vi "File Settings Dialog.vi"(8 "error in":errorcluster, 11 "Report Viewer in":refnum<class "Report Viewer.lvclass">) -> (0 "error out":errorcluster, 3 "Report Viewer out":refnum<class "Report Viewer.lvclass">)   [LabVIEW 2019, in "Report Viewer.lvlib" / "Report Viewer.lvclass"]
uses:
  Library/Report Viewer.lvclass
  Custom Controls/File Viewer Settings.ctl
  Custom Controls/Data Window.ctl
  Library/Report Viewer.lvclass/Report Viewer.ctl
  Custom Controls/Load Method.ctl
panel:
  in  "Default":bool caption="Cancel"
  in  "Cancel":bool
  in  "OK":bool caption="OK2"
  in  "File Navigation":enum32{"Number of Values", "By Time"}(tab)
  in  "Number of Values (graph)":T1={"Value Load"=enum."Load Selected", "Starting At"=0, "Number of Values"=100000}
  in  "Number of Values (table)":T1={"Value Load"=enum."Load Selected", "Starting At"=0, "Number of Values"=1000}
  in  "Data Window":T2 {"Seconds" max=60}
  # "Warning!  Setting the number of records too \nhigh can result in poor system performance"
  # "Warning!  Setting the number of records too \nhigh can result in poor system performance"
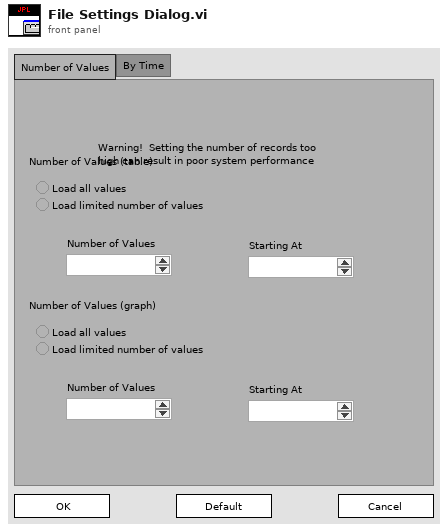
[diagram p1: front panel]
types:
  T1 = typedef "Report Viewer.lvlib/Report Viewer.lvclass/File Viewer Settings.ctl" = cluster{"Value Load":enum32{"Load All", "Load Selected"}, "Starting At":i32, "Number of Values":i32}
  T2 = typedef "Report Viewer.lvlib/Report Viewer.lvclass/Data Window.ctl" = cluster{"Data Start Time":timestamp, "Seconds":u32, "Minutes":u32, "Hours":u32}
  T3 = typedef "Report Viewer.lvlib/Report Viewer.lvclass/Load Method.ctl" = enum16{"Number of Values", "By Time"}
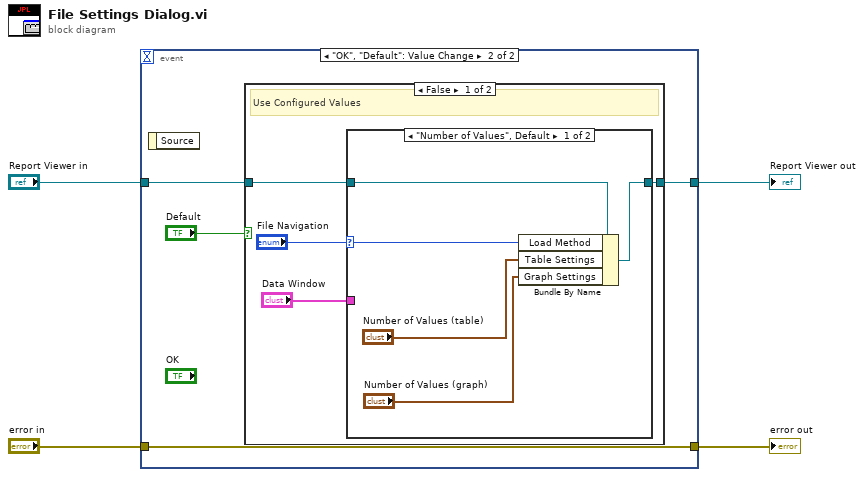
[diagram p0: block diagram]
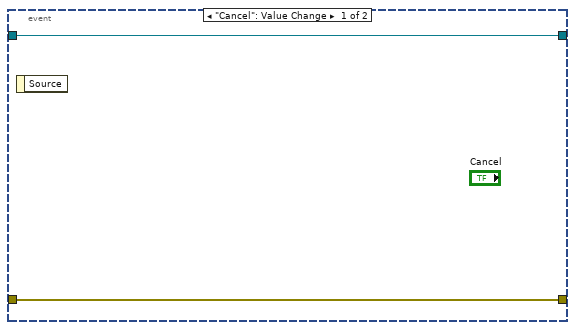
[diagram p2: hidden frame]
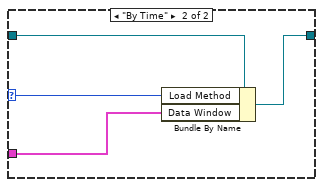
[diagram p3: hidden frame]
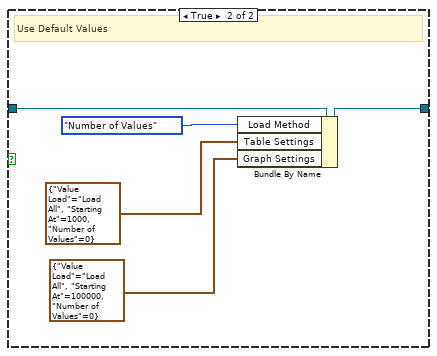
[diagram p4: hidden frame]
diagram:
  n1 = event shown="[1] \"OK\", \"Default\": Value Change" {
    selector: _ -> [_ _]
    dyn-events: _ -> [_ _]
    timeout: _ -> [_ _]
    tunnel: "Report Viewer in" -> [w6 w9]
    tunnel: [w6 w8] -> w3
    tunnel: [w5 w10] -> w2
    tunnel: "error in" -> [w5 w10]
    event "Cancel": Value Change {
      n2 = event-data() -> ()  [unwired: 1 in, 1 out]
    }
    event "OK", "Default": Value Change {
      n3 = event-data() -> ()  [unwired: 1 in, 1 out]
      n4 = case shown="False" "Default" {
        tunnel: w9 -> [w13 w28]
        tunnel: [w12 w27] -> w8
        frame False {
          # "Use Configured Values"
          n5 = case shown="\"Number of Values\", Default" "File Navigation" {
            selector: "File Navigation" -> [w17 w21]
            tunnel: w13 -> [w19 w23]
            tunnel: [w18 w22] -> w12
            tunnel: "Data Window" -> [_ w20]
            frame "Number of Values", Default {
              n6 = Bundle By Name(cluster=w19, "Load Method"=w17, "Table Settings"="Number of Values (table)", "Graph Settings"="Number of Values (graph)") -> (w18:refnum<class "Report Viewer.lvclass">)
            }
            frame "By Time" {
              n7 = Bundle By Name(cluster=w23, "Load Method"=w21, "Data Window"=w20) -> (w22:refnum<class "Report Viewer.lvclass">)
            }
          }
        }
        frame True {
          # "Use Default Values"
          n8 = Bundle By Name(cluster=w28, "Load Method"=Load_Method."Number of Values", "Table Settings"=T1 {"Value Load"=enum."Load All", "Starting At"=1000, "Number of Values"=0} ("File Viewer Settings"), "Graph Settings"=T1 {"Value Load"=enum."Load All", "Starting At"=100000, "Number of Values"=0} ("File Viewer Settings")) -> (w27:refnum<class "Report Viewer.lvclass">)
        }
      }
    }
  }
  "error out" <- w2
  "Report Viewer out" <- w3
